vi "Main_statistics.vi"() -> ()   [LabVIEW 2020]
uses:
  <vilib>/Analysis/NI_AALBase.lvlib
panel:
  in  "Tab Control":T1(tab)
  out "XYグラフ":T2(graph)
  in  "Select Mol Posi":u16(ring)=4 items=["3 molecules", "5 molecules", "7 molecules", "9 molecules", "13 molecules", "17 molecules", ""]
  out "Particle State":T3(array[cluster])
  in  "SD":dbl=0.11000000000000001
  in  "Tau_On":i32=40
  in  "Tau_Off":i32=10
  in  "Sim_Time":i32=100000
  in  "Asymmetry (X, Y)":dbl[](array[numeric])=[0.12000000000000001, 0.58]
  out "Count":i32
  in  "Torque 2":bool=TRUE
  in  "Torque":dbl=-24.0
  in  "停止":bool
  in  "Rot_Noise for Cargo":bool
  in  "Width of Rot_Noise":dbl format="%#_13g"
  out "Center State at T":T4
  out "iteration":i32
  in  "Iteration":i32=100
  in  "SaveFile":bool
  in  "Ini_Posi (3 mol)":dbl[][](array[numeric])=[[0.0, 0.0], [6.0, 0.0], [-6.0, 0.0]]
  in  "Ini_Posi (5 mol)":dbl[][](array[numeric])=[[0.0, 0.0], [6.0, 0.0], [-6.0, 0.0], [0.0, 6.0], [0.0, -6.0]]
  in  "Ini_Posi (9 mol)":dbl[][](array[numeric])=[[0.0, 0.0], [6.0, 0.0], [-6.0, 0.0], [0.0, 6.0], [0.0, -6.0], [6.0, 6.0], [6.0, -6.0], [-6.0, 6.0], [-6.0, -6.0]]
  in  "Ini_Posi (13 mol)":dbl[][](array[numeric])=[[0.0, 0.0], [6.0, 0.0], [-6.0, 0.0], [0.0, 6.0], [0.0, -6.0], [6.0, 6.0], [6.0, -6.0], [-6.0, 6.0], [-6.0, -6.0], [3.0, 3.0], [3.0, -3.0], [-3.0, 3.0], [-3.0, -3.0]]
  in  "Ini_Posi (13 mol#2)":dbl[][](array[numeric])=[[0.0, 0.0], [12.0, 3.0], [-12.0, 3.0], [12.0, -3.0], [-12.0, -3.0], [6.0, 0.0], [-6.0, 0.0], [0.0, -6.0], [0.0, 6.0], [6.0, 6.0], [6.0, -6.0], [-6.0, 6.0], [-6.0, -6.0], [3.0, 3.0], [3.0, -3.0], [-3.0, 3.0], [-3.0, -3.0]]
  in  "Ini_Posi (7 mol)":dbl[][](array[numeric])=[[0.0, 0.0], [5.0, 3.0], [-5.0, 3.0], [5.0, -3.0], [-5.0, -3.0], [0.0, 6.0], [0.0, -6.0]]
  out "N":i32
  out "mean":dbl caption="Mean_Y" format="%0.2f"
  out "standard deviation":dbl caption="SD_Y" format="%0.2f"
  out "mean 2":dbl caption="Mean_X" format="%0.2f"
  out "standard deviation 2":dbl caption="SD_X" format="%0.2f"
  out "N":i32
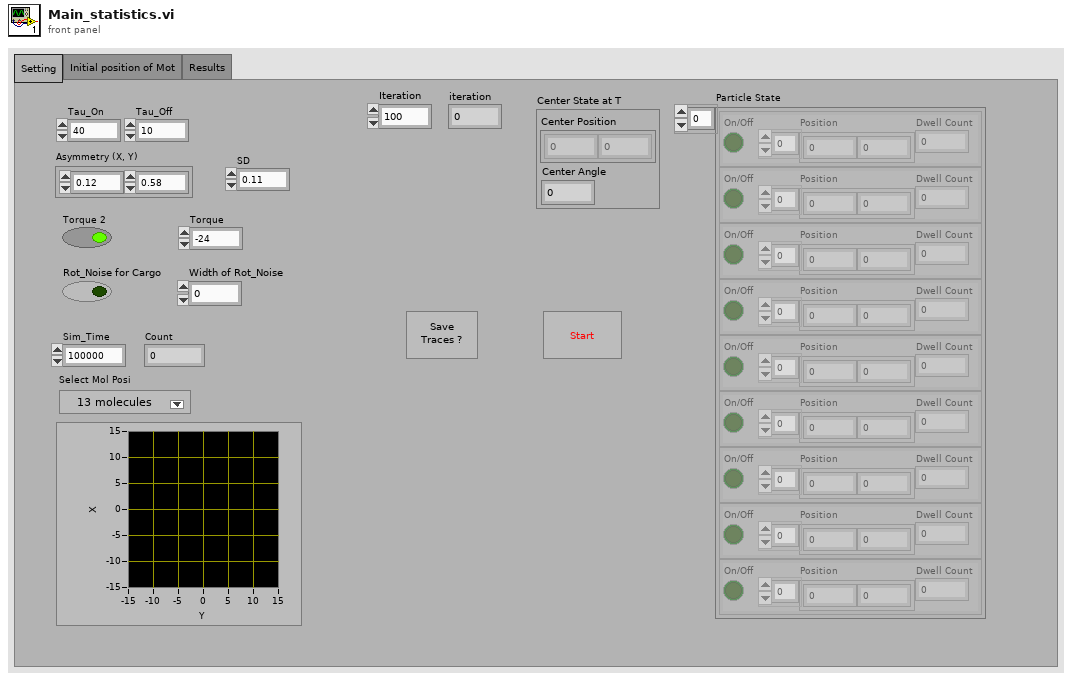
[diagram p1: front panel]
types:
  T1 = enum32{"Setting", "Initial position of Mot", "Results"}
  T2 = cluster{"Ini_Anchor_Posi (17 mol)":dbl[], "Ini_Anchor_Posi (17 mol)":dbl[]}
  T3 = cluster{"On/Off":bool, "Position":dbl[], "Dwell Count":i32}[]
  T4 = cluster{"Center Position":dbl[], "Center Angle":dbl}
  T5 = enum32{"Setting", "Initial position of Mot", "Results", "Results 2"}
  T6 = cluster{"Ini_Posi (13 mol#2)":dbl[], "Ini_Posi (13 mol#2)":dbl[]}
  T7 = cluster{"On/Off":bool, "Position":dbl[], "Next Dwell":i32}[]
  T8 = cluster{"On/Off":bool, "Position":dbl[], "Next Dwell":i32}
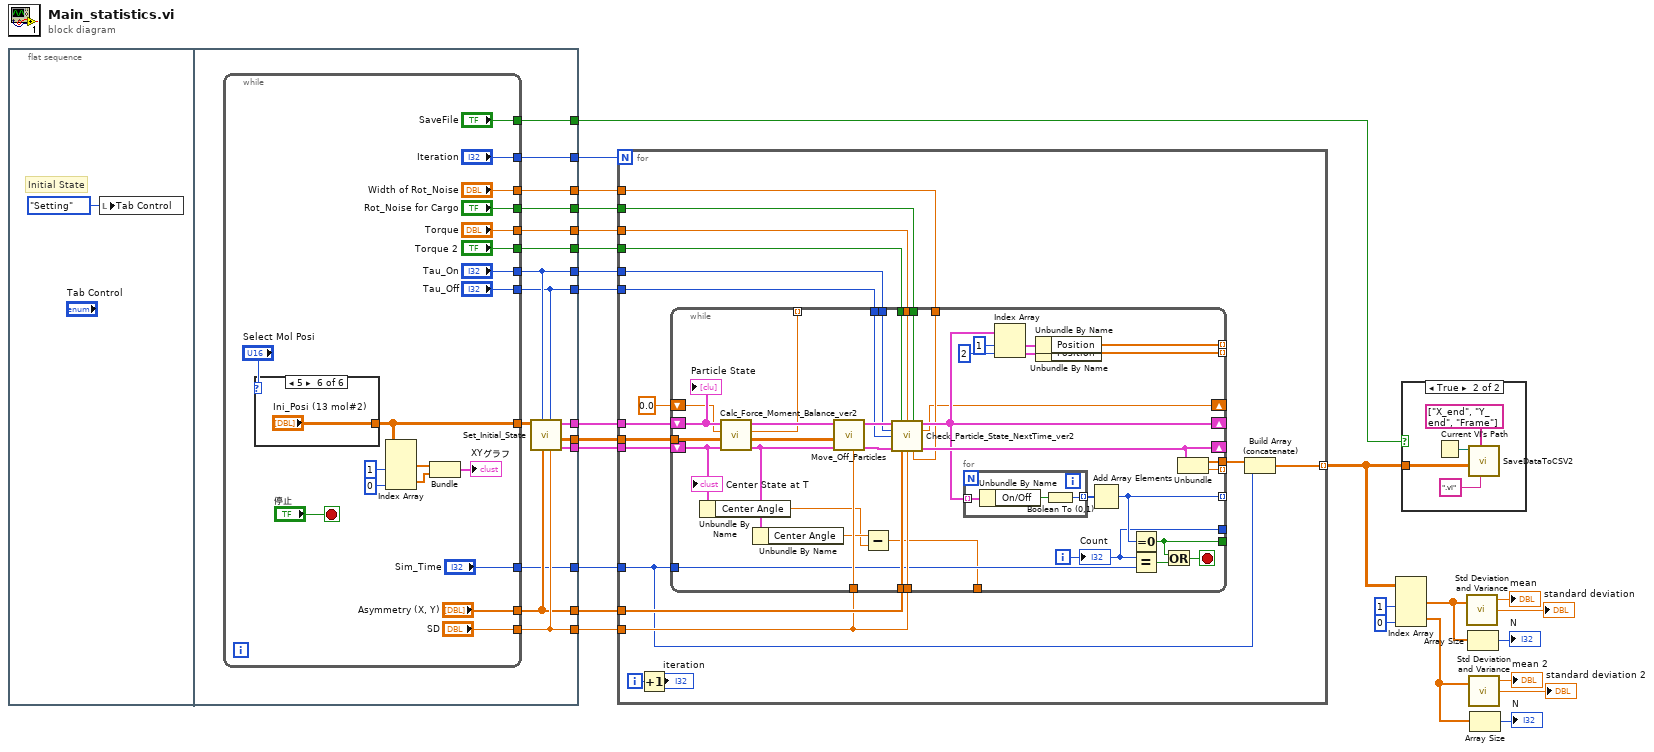
[diagram p0: block diagram]
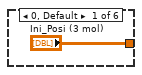
[diagram p3: hidden frame]
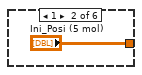
[diagram p4: hidden frame]
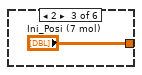
[diagram p5: hidden frame]
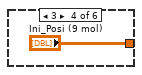
[diagram p6: hidden frame]
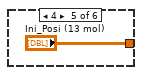
[diagram p7: hidden frame]
diagram:
  n1 = flat-sequence {
    tunnel: [w41] -> w25
    tunnel: [w40] -> w24
    tunnel: [w39] -> w23
    tunnel: [w36] -> w19
    tunnel: [w38] -> w22
    tunnel: [w37] -> w21
    tunnel: [w35] -> w20
    tunnel: [w34] -> w18
    tunnel: [w33] -> w17
    tunnel: [w31] -> w16
    tunnel: [w30] -> w15
    tunnel: [w29] -> w14
    tunnel: [w28] -> w2
    tunnel: [w27] -> w1
    frame #0 {
      # "Initial State"
      n2 = local write "Tab Control"(T5."Setting" ("Tab Control")) -> ()
    }
    frame #1 {
      n3 = while {
        tunnel: ["Tau_On"] -> w38
        tunnel: ["Tau_Off"] -> w37
        tunnel: ["SD"] -> w36
        tunnel: ["Asymmetry (X, Y)"] -> w35
        tunnel: ["Torque 2"] -> w34
        tunnel: ["Torque"] -> w33
        tunnel: [w54] -> w32
        tunnel: ["Rot_Noise for Cargo"] -> w31
        tunnel: ["Width of Rot_Noise"] -> w30
        tunnel: ["Sim_Time"] -> w29
        tunnel: ["Iteration"] -> w28
        tunnel: ["SaveFile"] -> w27
        stop <- "停止" stop-if-true
        n4 = case shown="5" "Select Mol Posi" {
          tunnel: ["Ini_Posi (3 mol)" "Ini_Posi (5 mol)" "Ini_Posi (7 mol)" "Ini_Posi (9 mol)" "Ini_Posi (13 mol)" "Ini_Posi (13 mol#2)"] -> w54
          frame 0, Default {
          }
          frame 1 {
          }
          frame 2 {
          }
          frame 3 {
          }
          frame 4 {
          }
          frame 5 {
          }
        }
        n5 = Index Array(array=w54, index (col) #1=1 ("無効な指標 (列)"), index (col) #2=0 ("指標 (列)")) -> (element #1=w49:dbl[], element #2=w48:dbl[])  [unwired: 2 in]
        n6 = Bundle("Ini_Posi (13 mol#2)"=w49, "Ini_Posi (13 mol#2)"=w48) -> (→"XYグラフ":T6)  [unwired: 1 in]
      }
      n7 = call "Set_Initial_State.vi"("SD"=w36, "Tau_Off"=w37, "Asymmetry (X, Y)"=w35, "Tau_On"=w38, "Ini_Anchor_Posi"=w32) -> ("Center State at T"=w39:T4, "Ini_Anchor_Posi"=w40:dbl[][], "On_Particle State"=w41:T3)  [unwired: 4 in]
    }
  }
  n8 = for {
    N: w2 -> [_]
    tunnel: w25 -> [w83]
    tunnel: w24 -> [w82]
    tunnel: w23 -> [w81]
    tunnel: w22 -> [w80]
    tunnel: w21 -> [w79]
    tunnel: w20 -> [w78]
    tunnel: w19 -> [w77]
    tunnel: w18 -> [w76]
    tunnel: w17 -> [w75]
    tunnel: w16 -> [w74]
    tunnel: w15 -> [w73]
    tunnel: w14 -> [w69]
    tunnel: [w68] -> w3 mode=indexing
    i -> [w71]
    n9 = Increment(x=w71) -> (x+1=→"iteration":i32)
    n10 = while {
      tunnel: w82 -> [w94]
      shift-right: [w115] -> _
      shift-left: w81 -> [w89]
      shift-right: [w107] -> _
      shift-left: w83 -> [w95]
      tunnel: w77 -> [w118]
      tunnel: w80 -> [w114]
      tunnel: w79 -> [w113]
      tunnel: w78 -> [w110]
      tunnel: [w121] -> _ mode=indexing
      tunnel: [w120] -> _ mode=indexing
      tunnel: [w119] -> w70
      tunnel: w77 -> [w109]
      tunnel: w76 -> [w111]
      tunnel: w75 -> [w112]
      tunnel: [w108] -> _ mode=indexing
      tunnel: [w102] -> _ mode=indexing
      tunnel: w69 -> [w103]
      tunnel: [w99] -> _
      tunnel: [w98] -> _
      tunnel: w74 -> [w97]
      tunnel: w73 -> [w96]
      shift-right: [w90] -> _
      shift-left: 0.0 ("Torque") -> [w91]
      tunnel: [w85] -> _
      tunnel: [w84] -> _ mode=indexing
      i -> [w98]
      stop <- w100 stop-if-true
      n11 = Unbundle By Name(w89) -> ("Center Angle"=w86:dbl)
      n12 = call "Calc_Force_Moment_Balance_ver2.vi"("Center State at T"=w89, "Ini_Anchor_Posi"=w94, "Torque"=w91, "On_Particle State"=w95) -> ("New Center State at T"=w88:T4, "Ini_Anchor_Posi"=w92:dbl[][], "Rot_angle"=w84:dbl, "On_Particle State"=w93:T3)  [unwired: 2 in, 2 out]
      n13 = Unbundle By Name(w88) -> ("Center Angle"=w87:dbl)
      n14 = call "Move_Off_Particles.vi"("SD"=w118, "Center State at T"=w88, "Ini_Anchor_Posi"=w92, "Particle Posi at T"=w93) -> ("Center State at T"=w116:T4, "New Particle Posi at T"=w117:T7)  [unwired: 6 in]
      n15 = Subtract(x=w87, y=w86) -> (x-y=w85:dbl)
      n16 = call "Check_Particle_State_NextTime_ver2.vi"("Particle State at T"=w117, "Torque?"=w111, "Torque"=w112, "Rot diffusion\nfor Cargo?"=w97, "Tau_On"=w114, "Tau_Off"=w113, "Center State at T"=w116, "Asymmetry (X, Y)"=w110, "SD"=w109, "Rot diffusion\nfor Cargo"=w96) -> ("Particle State at T+1"=w107:T7, "Torque"=w90:dbl, "New Center State at T"=w115:T4)  [unwired: 2 in, 1 out]
      n17 = for {
        tunnel: w107 -> [w126] mode=indexing
        tunnel: [w124] -> w106 mode=indexing
        n18 = Unbundle By Name(w126) -> ("On/Off"=w125:bool)
        n19 = Boolean To (0,1)(Boolean=w125) -> (0, 1=w124:i16)
      }
      n20 = Index Array(array=w107, index #1=1 ("index"), index #2=2 ("index")) -> (element #1=w123:T8, element #2=w122:T8)
      n21 = Unbundle By Name(w123) -> ("Position"=w121:dbl[])
      n22 = Unbundle By Name(w122) -> ("Position"=w120:dbl[])
      n23 = Add Array Elements(numeric array=w106) -> (sum=w102:i16)
      n24 = Equal To 0?(x=w102) -> (x = 0?=w99:bool)
      n25 = Equal?(x=w98, y=w103) -> (x = y?=w101:bool)
      n26 = Or(x=w99, y=w101) -> (x .or. y?=w100:bool)
      n27 = Unbundle(w115) -> ("Center Position"=w119:dbl[], "Center Angle"=w108:dbl)
      "Particle State" <- w95
      "Count" <- w98
      "Center State at T" <- w89
    }
    n28 = Build Array (concatenate)(w70, w69) -> (w68:dbl[])
  }
  n29 = Index Array(array=w3, index (col) #1=1 ("無効な指標 (列)"), index (col) #2=0 ("指標 (列)")) -> (element #1=w10:dbl[], element #2=w4:dbl[])  [unwired: 2 in]
  n30 = case shown="TRUE" w1 {
    tunnel: w3 -> [_ w129]
    frame False {
    }
    frame True {
      n31 = Current VI's Path() -> (path=w128:path)
      n32 = call "SaveDataToCSV2.vi"("OmitFileName"=".vi", "Header"=string[] ["X_end", "Y_end", "Frame"], "Data"=w129, "パス"=w128) -> ()  [unwired: 8 in]
    }
  }
  n33 = call <vilib>:"Std Deviation and Variance.vi"("X"=w10) -> ("mean"=→"mean":dbl, "standard deviation"=→"standard deviation":dbl)  [unwired: 1 in, 1 out]
  n34 = Array Size(array=w10) -> (size(s)=→"N":i32)
  n35 = call <vilib>:"Std Deviation and Variance.vi"("X"=w4) -> ("mean"=→"mean 2":dbl, "standard deviation"=→"standard deviation 2":dbl)  [unwired: 1 in, 1 out]
  n36 = Array Size(array=w4) -> (size(s)=→"N":i32)
